vi "Generate_SC.vi"(6 "A":dbl=15000.0, 8 "error in (no error)":errorcluster, 9 "pos":dbl=550.0 format="%#_13g", 10 "Type of signal":string="BG", 11 "Emulate in":refnum<class "Emulate.lvclass">) -> (0 "error out":errorcluster, 2 "SC output":i32[](array[numeric]), 3 "Emulate out":refnum<class "Emulate.lvclass">)   [LabVIEW 2015, in "Emulate.lvclass"]
uses:
  Emulate.lvclass
  Detector.lvclass/Detector.ctl
  Detector.lvclass
panel:
  in  "error sig/ref":dbl=0.001 format="%#_13g"
  in  "sigma":dbl=85.0 format="%#_13g"
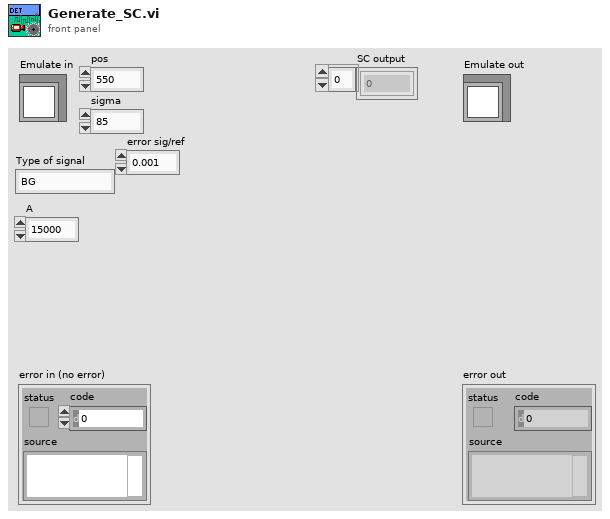
[diagram p1: front panel]
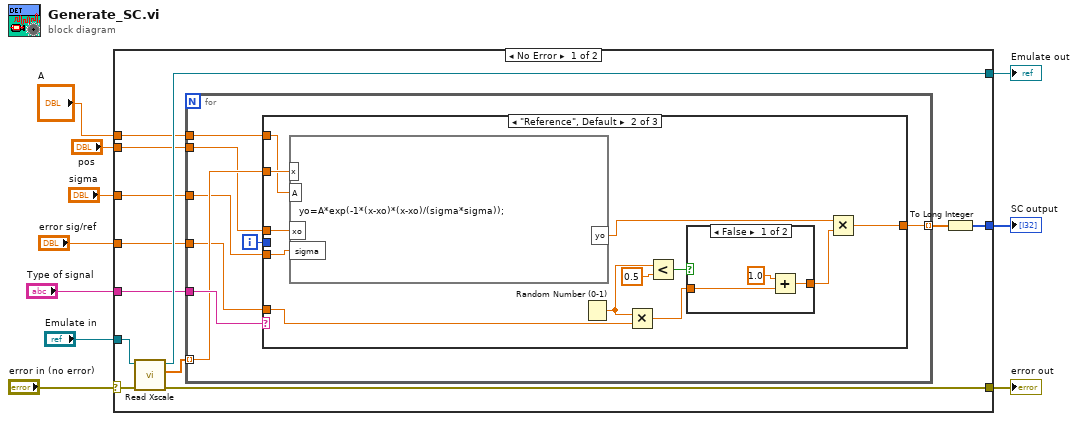
[diagram p0: block diagram]
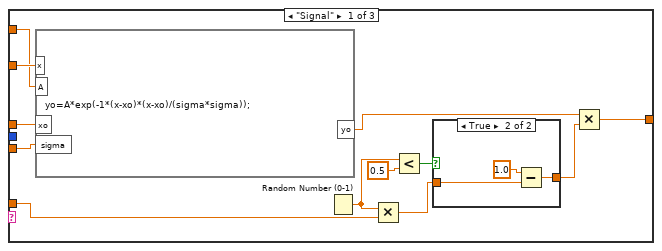
[diagram p2: hidden frame]
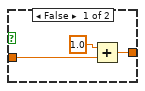
[diagram p3: hidden frame]
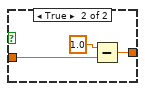
[diagram p4: hidden frame]
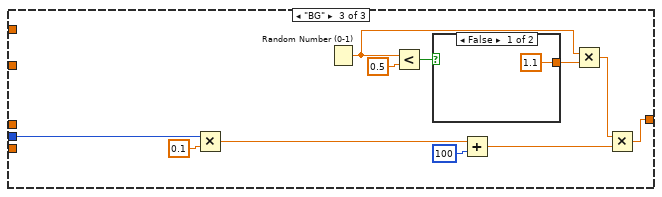
[diagram p5: hidden frame]
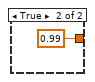
[diagram p6: hidden frame]
diagram:
  n1 = case shown="No Error" "error in (no error)" {
    selector: "error in (no error)" -> [w21 w81]
    tunnel: [w15 w81] -> w9
    tunnel: [w20 w80] -> w7
    tunnel: "Emulate in" -> [w22 w80]
    tunnel: [w17 _] -> w6
    tunnel: "Type of signal" -> [w16 _]
    tunnel: "pos" -> [w14 _]
    tunnel: "sigma" -> [w13 _]
    tunnel: "error sig/ref" -> [w12 _]
    tunnel: "A" -> [w11 _]
    frame No Error {
      n2 = call "Read Xscale.vi"("error in (no error)"=w21, "Detector en entrée"=w22) -> ("error out"=w15:errorcluster, "Xscale"=w19:dbl[], "Detector en sortie"=w20:refnum<class "Emulate.lvclass">)  [unwired: 7 in]
      n3 = for {
        tunnel: w19 -> [w27] mode=indexing
        tunnel: [w30] -> w18 mode=indexing
        tunnel: w16 -> [w29]
        tunnel: w14 -> [w26]
        tunnel: w13 -> [w25]
        tunnel: w12 -> [w24]
        tunnel: w11 -> [w23]
        i -> [w28]
        n4 = case shown="\"Reference\", Default" w29 {
          tunnel: [w41 w60 w67] -> w30
          tunnel: w28 -> [_ _ w72]
          tunnel: w27 -> [w39 w56 _]
          tunnel: w26 -> [w38 w57 _]
          tunnel: w25 -> [w37 w55 _]
          tunnel: w24 -> [w34 w52 _]
          tunnel: w23 -> [w31 w49 _]
          frame "Signal" {
            n5 = formula code="yo=A*exp(-1*(x-xo)*(x-xo)/(sigma*sigma));"("xo"=w38, "sigma"=w37, "x"=w39, "A"=w31) -> ("yo"=w42:dbl)
            n6 = Random Number (0-1)() -> (number: 0 to 1=w35:dbl)
            n7 = Multiply(x=w35, y=w34) -> (x*y=w33:dbl)
            n8 = Less?(x=w35, y=0.5) -> (x < y?=w36:bool)
            n9 = case shown="True" w36 {
              tunnel: [w44 w47] -> w32
              tunnel: w33 -> [w43 w46]
              frame False {
                n10 = Add(x=1.0, y=w43) -> (x+y=w44:dbl)
              }
              frame True {
                n11 = Subtract(x=1.0, y=w46) -> (x-y=w47:dbl)
              }
            }
            n12 = Multiply(x=w42, y=w32) -> (x*y=w41:dbl)
          }
          frame "Reference", Default {
            n13 = formula code="yo=A*exp(-1*(x-xo)*(x-xo)/(sigma*sigma));"("xo"=w57, "sigma"=w55, "x"=w56, "A"=w49) -> ("yo"=w54:dbl)
            n14 = Random Number (0-1)() -> (number: 0 to 1=w51:dbl)
            n15 = Multiply(x=w51, y=w52) -> (x*y=w50:dbl)
            n16 = Less?(x=w51, y=0.5) -> (x < y?=w58:bool)
            n17 = case shown="False" w58 {
              tunnel: [w61 w64] -> w53
              tunnel: w50 -> [w62 w66]
              frame False {
                n18 = Add(x=1.0, y=w62) -> (x+y=w61:dbl)
              }
              frame True {
                n19 = Subtract(x=1.0, y=w66) -> (x-y=w64:dbl)
              }
            }
            n20 = Multiply(x=w54, y=w53) -> (x*y=w60:dbl)
          }
          frame "BG" {
            n21 = Multiply(x=w72, y=0.1) -> (x*y=w71:dbl)
            n22 = Random Number (0-1)() -> (number: 0 to 1=w74:dbl)
            n23 = Less?(x=w74, y=0.5) -> (x < y?=w76:bool)
            n24 = case shown="False" w76 {
              tunnel: [1.1 ("y") 0.99 ("y")] -> w75
              frame False {
              }
              frame True {
              }
            }
            n25 = Add(x=w71, y=100) -> (x+y=w69:dbl)
            n26 = Multiply(x=w74, y=w75) -> (x*y=w68:dbl)
            n27 = Multiply(x=w68, y=w69) -> (x*y=w67:dbl)
          }
        }
      }
      n28 = To Long Integer(number=w18) -> (32bit integer=w17:i32[])
    }
    frame Error {
    }
  }
  "error out" <- w9
  "Emulate out" <- w7
  "SC output" <- w6
